vi "Controlcenter.vi"() -> ()   [LabVIEW 2010]
uses:
  glob_var.vi
  robo_interface_distribute/Robo Interface/Advanced/_Close/_Comm/Close Device Comm.vi
panel:
  out "lichtstatus":bool=TRUE
  in  "new_target":i32
  in  "beenden":bool
  out "Device ID Out":T1(ring)
  in  "stop":bool
  in  "end":bool
  in  "autom-auswahl":bool=TRUE caption="Auswahlautom"
  in  "automatisch":bool=TRUE caption="Autom. Betrieb"
  in  "licht":bool
  in  "baustein-einzug":bool
  out "log":string caption="Log"
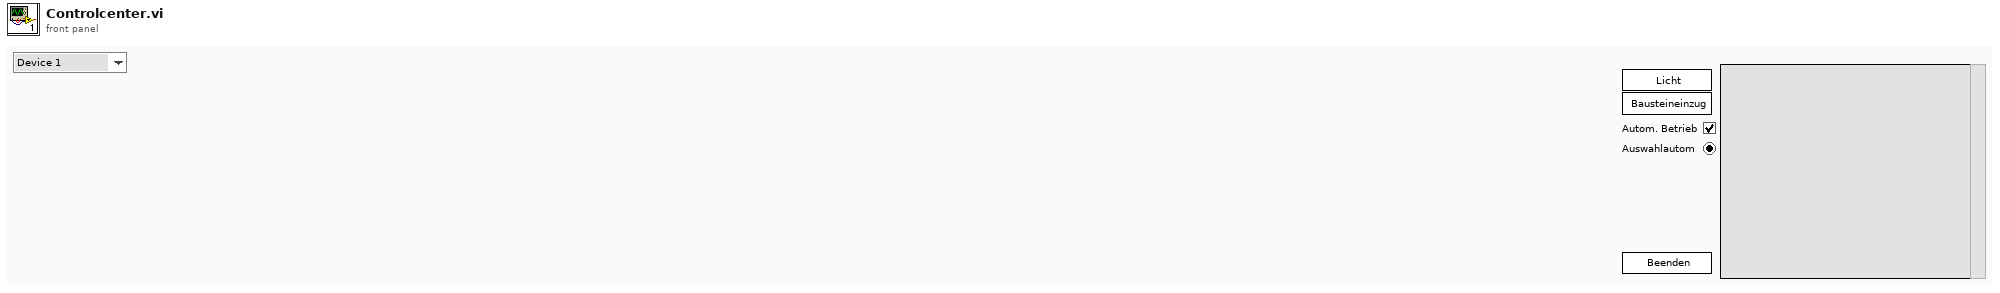
[diagram p1: front panel]
types:
  T1 = enum16{"Device 1", "Device 2", "Device 3", "Device 4", "Device 5", "Device 6", "Device 7", "Device 8"}
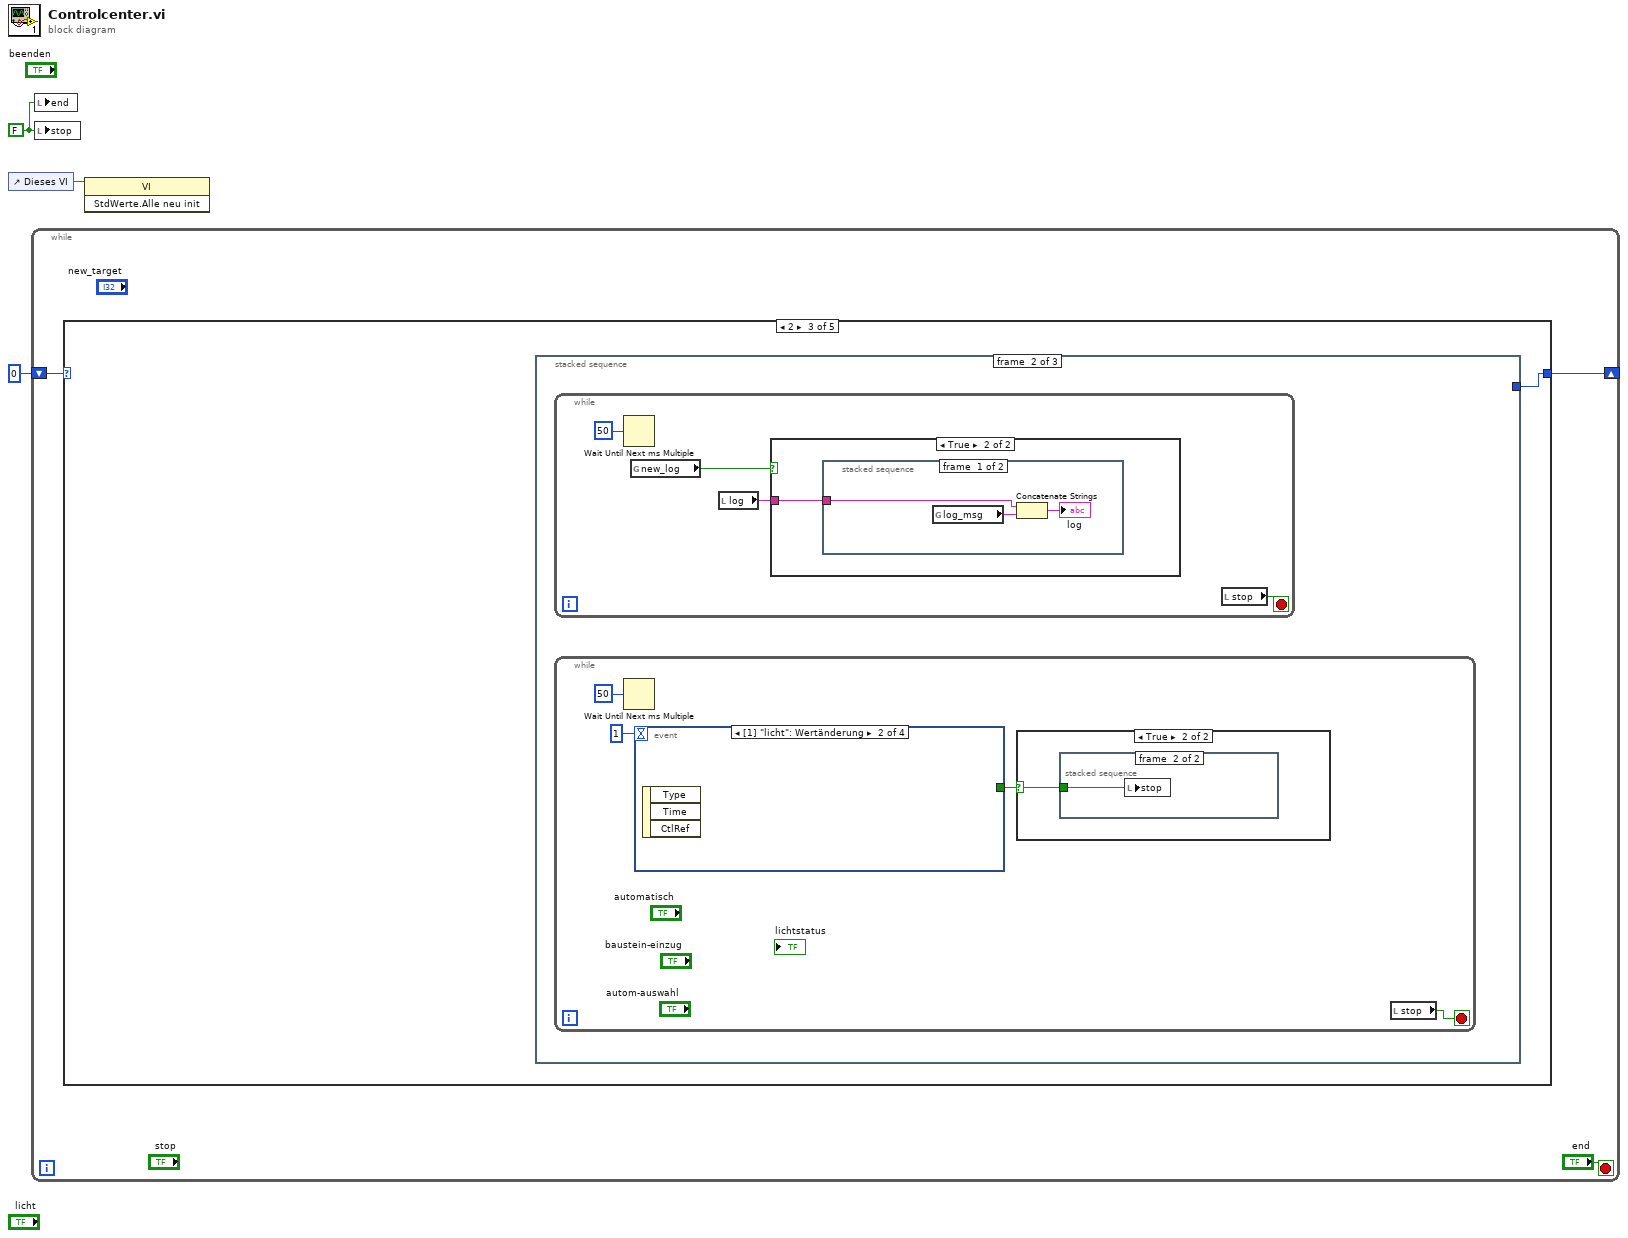
[diagram p0: block diagram]
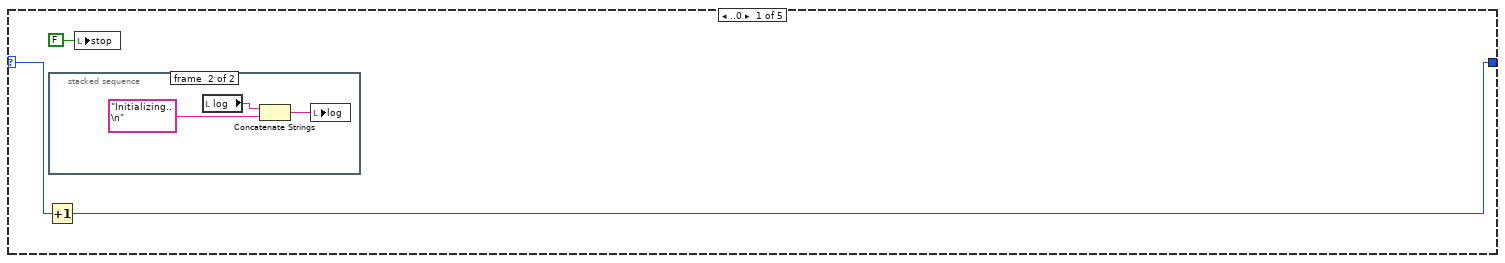
[diagram p2: hidden frame]
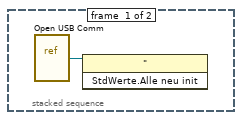
[diagram p3: hidden frame]
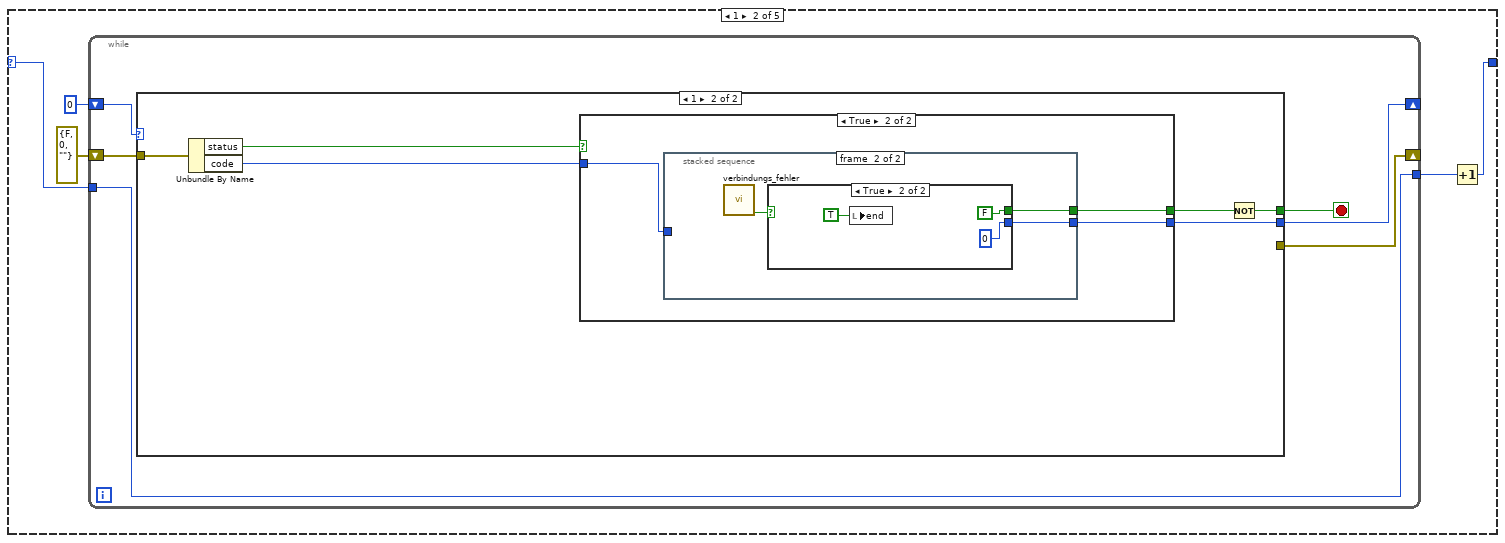
[diagram p4: hidden frame]
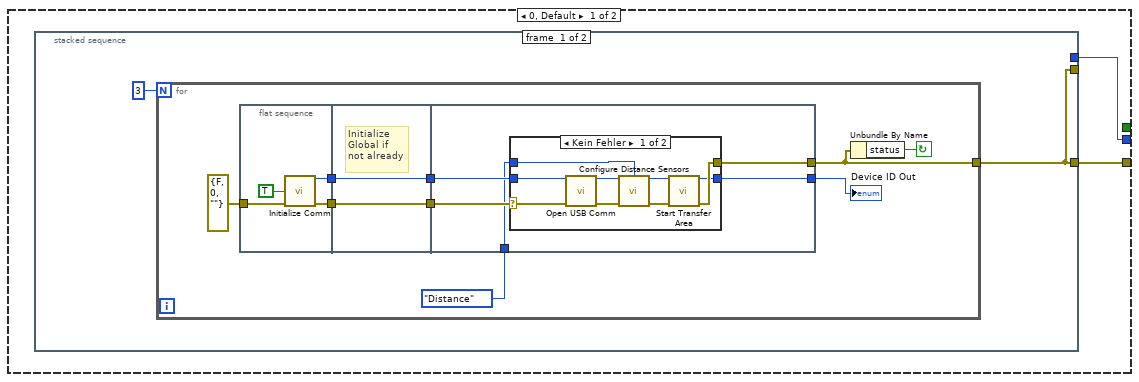
[diagram p5: hidden frame]
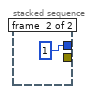
[diagram p7: hidden frame]
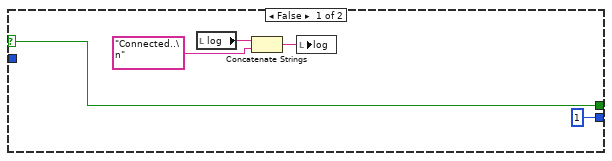
[diagram p8: hidden frame]
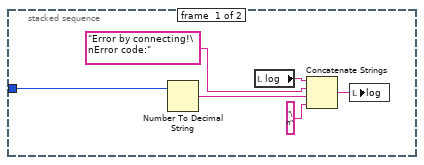
[diagram p9: hidden frame]
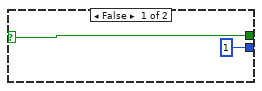
[diagram p10: hidden frame]
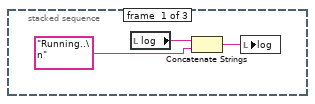
[diagram p11: hidden frame]
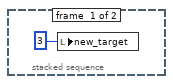
[diagram p13: hidden frame]
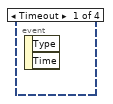
[diagram p14: hidden frame]
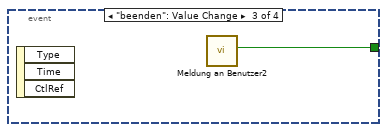
[diagram p15: hidden frame]
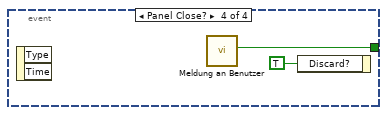
[diagram p16: hidden frame]
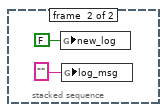
[diagram p18: hidden frame]
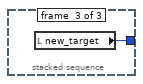
[diagram p19: hidden frame]
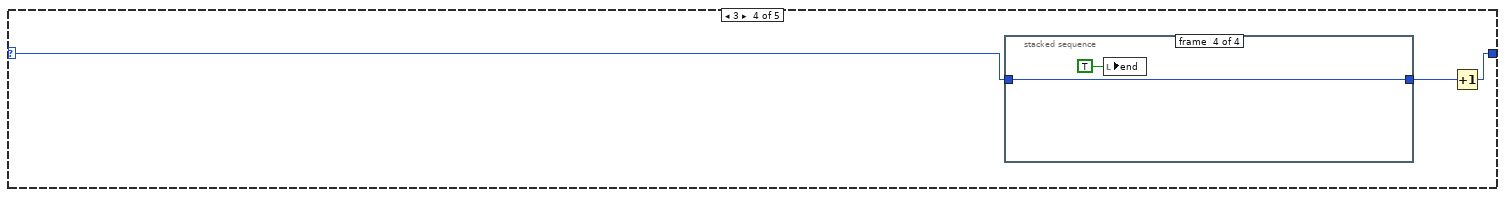
[diagram p20: hidden frame]
diagram:
  w1 = FALSE
  n1 = control-ref of="Dieses VI"() -> (w2:refnum<vi>)
  n2 = while {
    shift-right: [w4] -> _
    shift-left: 0 -> [w5]
    stop <- "end" stop-if-true
    n3 = case shown="2" w5 {
      selector: w5 -> [w8 w16 _ w115 w128]
      tunnel: [w7 w14 w89 w116 w128] -> w4
      frame ..0 {
        n4 = Increment(x=w8) -> (x+1=w7:i32)
        n5 = stacked-sequence {
          frame #0 {
            n6 = vi-ref "Open USB Comm.vi"() -> (w10:refnum<vi>)
            n7 = invoke class="\"" method="StdWerte.Alle neu init"(reference=w10) -> ()  [unwired: 2 in, 3 out]
          }
          frame #1 {
            n8 = local read "log"() -> (w11:string)
            n9 = Concatenate Strings(w11, "Initializing..\n") -> (w13:string)
            n10 = local write "log"(w13) -> ()
          }
        }
        n11 = local write "stop"(FALSE ("stop")) -> ()
      }
      frame 1 {
        n12 = while {
          shift-right: [w23] -> _
          shift-left: 0 -> [w24]
          shift-right: [w22] -> _
          shift-left: errorcluster {"status"=FALSE, "code"=0, "source"=""} ("error IO") -> [w21]
          tunnel: w16 -> [w19]
          tunnel: [w19] -> w15
          stop <- w20 stop-if-true
          n13 = case shown="1" w24 {
            tunnel: [w26 w61] -> w23
            tunnel: [w25 _] -> w22
            tunnel: w21 -> [_ w66]
            tunnel: [_ w64] -> w20
            frame 0, Default {
              n14 = stacked-sequence {
                tunnel: [_ 1] -> w26
                tunnel: [w27 _] -> _
                tunnel: [w27 _] -> w25
                frame #0 {
                  n15 = for {
                    N: 3 -> [_]
                    tunnel: [w30] -> w27
                    stop <- w29 continue-if-true
                    n16 = flat-sequence {
                      tunnel: [w41] -> w37
                      tunnel: [w40] -> w36
                      tunnel: errorcluster {"status"=FALSE, "code"=0, "source"=""} ("error in") -> [w39]
                      tunnel: [w43] -> w35
                      tunnel: [w42] -> w34
                      tunnel: w37 -> [w43]
                      tunnel: w36 -> [w42]
                      tunnel: w35 -> [w48]
                      tunnel: w34 -> [w47]
                      tunnel: [w46] -> w30
                      tunnel: [w45] -> w33
                      tunnel: enum32{"Voltage", "Distance"}."Distance" ("Distance Sensor Mode") -> [w44]
                      frame #0 {
                        n17 = call "Initialize Comm.vi"("immer erster aufruf?"=TRUE, "error in"=w39) -> ("Device ID Out"=w41:T1, "error out"=w40:errorcluster)  [unwired: 1 in, 11 out]
                      }
                      frame #1 {
                        # "Initialize\nGlobal if\nnot already"
                      }
                      frame #2 {
                        n18 = case shown="Kein Fehler" w47 {
                          selector: w47 -> [w54 w59]
                          tunnel: [w57 w59] -> w46
                          tunnel: w48 -> [w52 w58]
                          tunnel: [w56 w58] -> w45
                          tunnel: w44 -> [w50 _]
                          frame No Error {
                            n19 = call "Open USB Comm.vi"("Device ID"=w52, "error in"=w54) -> ("Device ID Out"=w51:T1, "error out"=w53:errorcluster)  [unwired: 12 out]
                            n20 = call "Configure Distance Sensors.vi"("Device ID"=w51, "Distance Sensor Mode"=w50, "error in"=w53) -> ("Device ID Out"=w49:T1, "error out"=w55:errorcluster)  [unwired: 6 in, 5 out]
                            n21 = call "Start Transfer Area.vi"("Device ID"=w49, "error in"=w55) -> ("Device ID Out"=w56:T1, "error out"=w57:errorcluster)  [unwired: 12 out]
                          }
                          frame Error {
                          }
                        }
                      }
                    }
                    n22 = Unbundle By Name(w30) -> ("status"=w29:bool)
                    "Device ID Out" <- w33
                  }
                }
                frame #1 {
                }
              }
            }
            frame 1 {
              n23 = Unbundle By Name(w66) -> ("status"=w65:bool, "code"=w63:i32)
              n24 = case shown="True" w65 {
                selector: w65 -> [w68 _]
                tunnel: w63 -> [_ w74]
                tunnel: [w68 w72] -> w62
                tunnel: [1 w73] -> w61
                frame False {
                  n25 = local read "log"() -> (w71:string)
                  n26 = Concatenate Strings(w71, "Connected..\n" ("String")) -> (w69:string)
                  n27 = local write "log"(w69) -> ()
                }
                frame True {
                  n28 = stacked-sequence {
                    tunnel: w74 -> [w79 _]
                    tunnel: [_ w83] -> w73
                    tunnel: [_ w81] -> w72
                    frame #0 {
                      n29 = Number To Decimal String(number=w79) -> (decimal integer string=w78:string)  [unwired: 1 in]
                      n30 = local read "log"() -> (w76:string)
                      n31 = Concatenate Strings(w76, "Error by connecting!\nError code:", w78, "\n" ("String")) -> (w77:string)
                      n32 = local write "log"(w77) -> ()
                    }
                    frame #1 {
                      n33 = call "verbindungs_fehler.vi"() -> ("schließen?"=w82:bool)  [unwired: 11 in]
                      n34 = case shown="True" w82 {
                        selector: w82 -> [w84 _]
                        tunnel: [1 0] -> w83
                        tunnel: [w84 FALSE] -> w81
                        frame False {
                        }
                        frame True {
                          n35 = local write "end"(TRUE ("end")) -> ()
                        }
                      }
                    }
                  }
                }
              }
              n36 = Not(x=w62) -> (.not. x?=w64:bool)
            }
          }
        }
        n37 = Increment(x=w15) -> (x+1=w14:i32)
      }
      frame 2 {
        n38 = stacked-sequence {
          tunnel: [_ _ w113] -> w89
          frame #0 {
            n39 = local read "log"() -> (w91:string)
            n40 = Concatenate Strings(w91, "Running..\n" ("String")) -> (w90:string)
            n41 = local write "log"(w90) -> ()
          }
          frame #1 {
            n42 = while {
              stop <- w103 stop-if-true
              n43 = Wait Until Next ms Multiple(millisecond multiple=u32 50 ("Vielfache von ms")) -> ()  [unwired: 1 out]
              n44 = global read "glob_var.vi" "new_log"() -> (w105:bool)
              n45 = local read "log"() -> (w104:string)
              n46 = case shown="True" w105 {
                tunnel: w104 -> [_ w107]
                frame False {
                }
                frame True {
                  n47 = stacked-sequence {
                    tunnel: w107 -> [w110 _]
                    frame #0 {
                      n48 = global read "glob_var.vi" "log_msg"() -> (w109:string)
                      n49 = Concatenate Strings(w110, w109) -> (→"log":string)
                    }
                    frame #1 {
                      n50 = global write "glob_var.vi" "new_log"(FALSE ("new_log")) -> ()
                      n51 = global write "glob_var.vi" "log_msg"("" ("log_msg")) -> ()
                    }
                  }
                }
              }
              n52 = local read "stop"() -> (w103:bool)
            }
            n53 = while {
              stop <- w94 stop-if-true
              n54 = Wait Until Next ms Multiple(millisecond multiple=u32 50 ("Vielfache von ms")) -> ()  [unwired: 1 out]
              n55 = event shown="[1] \"licht\": Wertänderung" {
                selector: _ -> [_ _ _ _]
                dyn-events: _ -> [_ _ _ _]
                timeout: 1 -> [_ _ _ _]
                tunnel: [_ _ w100 w101] -> w93
                event Timeout {
                  n56 = event-data() -> ()  [unwired: 1 in, 2 out]
                }
                event "licht": Value Change {
                  n57 = event-data() -> ()  [unwired: 1 in, 3 out]
                }
                event "beenden": Value Change {
                  n58 = event-data() -> ()  [unwired: 1 in, 3 out]
                  n59 = call "Meldung an Benutzer2"() -> ("Beenden"=w100:bool)  [unwired: 10 in, 1 out]
                }
                event Panel Close? {
                  n60 = event-data() -> ()  [unwired: 1 in, 2 out]
                  n61 = call "Meldung an Benutzer"() -> ("Beenden"=w101:bool)  [unwired: 10 in, 1 out]
                  n62 = event-data("Discard?"=TRUE ("Verwerfen?")) -> ()  [unwired: 1 in, 1 out]
                }
              }
              n63 = case shown="True" w93 {
                selector: w93 -> [_ w97]
                frame False {
                }
                frame True {
                  n64 = stacked-sequence {
                    tunnel: w97 -> [_ w99]
                    frame #0 {
                      n65 = local write "new_target"(3 ("new_target")) -> ()
                    }
                    frame #1 {
                      n66 = local write "stop"(w99) -> ()
                    }
                  }
                }
              }
              n67 = local read "stop"() -> (w94:bool)
            }
          }
          frame #2 {
            n68 = local read "new_target"() -> (w113:i32)
          }
        }
      }
      frame 3 {
        n69 = stacked-sequence {
          tunnel: w115 -> [_ _ _ w123]
          tunnel: [_ _ _ w123] -> w114
          frame #0 {
            n70 = local read "log"() -> (w119:string)
            n71 = Concatenate Strings(w119, "Disconnecting..\n" ("String")) -> (w117:string)
            n72 = local write "log"(w117) -> ()
          }
          frame #1 {
            n73 = call-poly "Close Comm.vi"() -> ()  [unwired: 2 in, 14 out]
          }
          frame #2 {
            n74 = local read "log"() -> (w122:string)
            n75 = Concatenate Strings(w122, "Stopping..\n" ("String")) -> (w120:string)
            n76 = local write "log"(w120) -> ()
          }
          frame #3 {
            n77 = local write "end"(TRUE ("end")) -> ()
          }
        }
        n78 = Increment(x=w114) -> (x+1=w116:i32)
      }
      frame 4.. {
        n79 = local read "log"() -> (w126:string)
        n80 = Concatenate Strings(w126, "Outrunning.." ("String")) -> (w127:string)
        n81 = local write "log"(w127) -> ()
      }
    }
  }
  n82 = local write "end"(w1) -> ()
  n83 = local write "stop"(w1) -> ()
  n84 = invoke class="VI" method="StdWerte.Alle neu init"(reference=w2) -> ()  [unwired: 2 in, 3 out]
